vi "Folder fit WLC.vi"() -> ()   [LabVIEW 2014]
uses:
  SubVI/WLC-Fitting Cluster.ctl
  <vilib>/Utility/file.llb/Write To Spreadsheet File (DBL).vi
  <vilib>/Analysis/NI_AALBase.lvlib
panel:
  out "mean K":dbl format="%0.2f"
  out "Lp-Time":cluster{i32[], "best fit parameters":dbl[]}(graph)
  out "Lc-Time":cluster{i32[], "best fit parameters":dbl[]}(graph)
  out "median Lc":dbl format="%0.2f"
  out "median Lp":dbl format="%0.2f"
  in  "Save?":bool
  in  "Enum":T1(ring)
  out "STD Lc":dbl format="%0.2f"
  out "STD Lp":dbl format="%0.2f"
  in  "DataRecord type":enum32{"OneDirectionOnly?", "TwoSide Data"}(tab)=enum."TwoSide Data"
  out "OneDirectionOnly?":bool=TRUE
  in  "Fit \"+\"(RHS) ?":bool=TRUE
  in  "Fit One Side?":bool
  out "r^2 Array":dbl[](array[numeric])
  out "mean Lc":dbl format="%0.2f"
  out "mean Lp":dbl format="%0.2f"
  out "Lc array":dbl[](array[numeric])
  out "Lp array":dbl[](array[numeric])
  out "best fit parameters":dbl[][](array[numeric])
  in  "Fitting Cluster":T2={"cr (um)"=0.0, "yr (V)"=0.0, "trap height(nm)"=300.0, "bead radius(nm)"=515.0, "Length offset"=550.0, "Upper Force(pN)"=500.0, "cr shift (nm)"=0.0, "yr shift (mV)"=0.0, "LaserPower (mW)"=1000.0, "conversion factor (V/um)"=0.0, "Stiffness (pN/nm)"=0.0, "xDNA cut outside"=3000.0, "Lower Force(pN)"=5.0, "c for zbd"=0.002}
  in  "initial parameters (Lp,Lc) or (Lc,K)":dbl[](array[numeric])=[40.0, 1150.0]
  in  "Folder Path":path
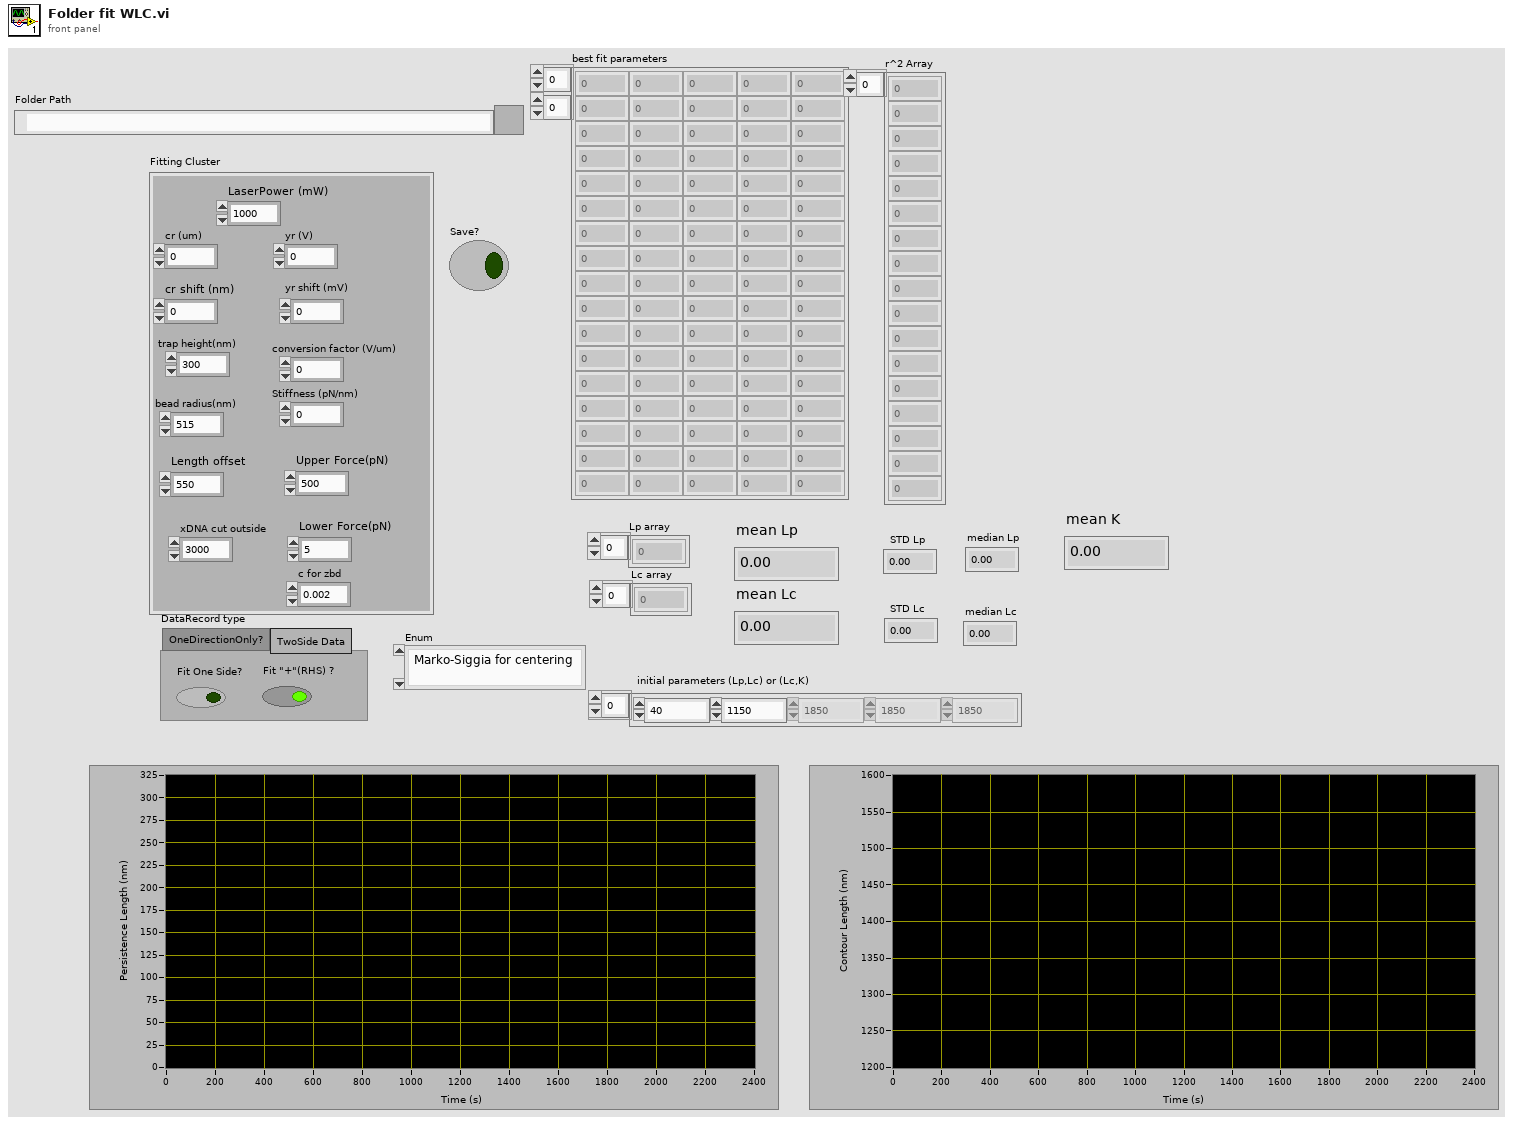
[diagram p1: front panel]
types:
  T1 = enum16{" Marko-Siggia for centering", "Marko-Siggia", "direct fit (Lp,Lc,K)", "fit K (Lp,Lc,K)", "eWLC (Lp=45,Lc,K)"}
  T2 = typedef "WLC-Fitting Cluster.ctl" = cluster{"cr (um)":dbl, "yr (V)":dbl, "trap height(nm)":dbl, "bead radius(nm)":dbl, "Length offset":dbl, "Upper Force(pN)":dbl, "cr shift (nm)":dbl, "yr shift (mV)":dbl, "LaserPower (mW)":dbl, "conversion factor (V/um)":dbl, "Stiffness (pN/nm)":dbl, "xDNA cut outside":dbl, "Lower Force(pN)":dbl, "c for zbd":dbl}
  T3 = cluster{"Time past (s)":i32[], "best fit parameters":dbl[]}
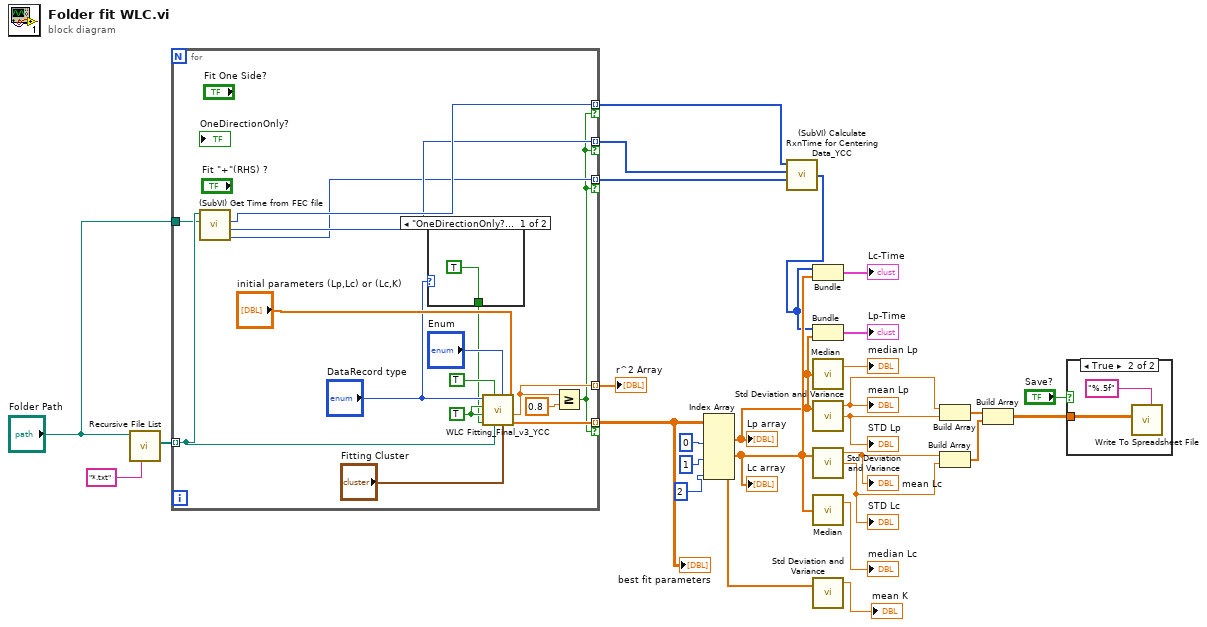
[diagram p0: block diagram]
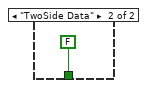
[diagram p3: hidden frame]
diagram:
  n1 = call <vilib>:"Recursive File List.vi"("pattern"="*.txt", "Folder Path"="Folder Path") -> ("All Files in Dir"=w27:path[])  [unwired: 5 in, 4 out]
  n2 = for {
    tunnel: w27 -> [w35] mode=indexing
    tunnel: [w41] -> w4 mode=indexing if=w30
    tunnel: [w39] -> w24 mode=indexing
    tunnel: "Folder Path" -> [w34]
    tunnel: [w33] -> w8 mode=indexing if=w30
    tunnel: [w32] -> w7 mode=indexing if=w30
    tunnel: [w31] -> w6 mode=indexing if=w30
    w44 = TRUE ("Ready to Fit")
    n3 = call "(SubVI) Get Time from FEC file.vi"("Folder path"=w34, "path"=w35) -> ("sec"=w31:i32, "min"=w32:i32, "hr"=w33:i32)  [unwired: 2 in, 1 out]
    n4 = case shown="\"OneDirectionOnly?\", Default" "DataRecord type" {
      tunnel: [TRUE ("T=Fit U or twoside\nF=Fit F") FALSE ("Save Calibrated Data?")] -> w29
      frame "OneDirectionOnly?", Default {
      }
      frame "TwoSide Data" {
      }
    }
    n5 = call "WLC Fitting_Final_v3_YCC.vi"("initial parameters (Lp,Lc) or (Lc,K)"="initial parameters (Lp,Lc) or (Lc,K)", "Fitting Cluster"="Fitting Cluster", "Enum"="Enum", "Load Stage-QPD data"=w35, "T=Fit U or twoside\nF=Fit F"=TRUE ("T=Fit U or twoside\nF=Fit F"), "F+U data?"=w29, "Finish Fitting"=w44, "Ready to Fit"=w44, "DataRecord type"="DataRecord type") -> ("best fit parameters"=w41:dbl[], "r^2"=w39:dbl)  [unwired: 1 in]
    n6 = Greater Or Equal?(x=w39, y=0.8) -> (x >= y?=w30:bool)
  }
  "best fit parameters" <- w4
  "r^2 Array" <- w24
  n7 = Index Array(array=w4, index (col) #1=0 ("disabled index (col)"), index (col) #2=1 ("disabled index (col)"), index (col) #3=2 ("disabled index (col)")) -> (element #1=w10:dbl[], element #2=w13:dbl[], element #3=w2:dbl[])  [unwired: 3 in]
  "Lp array" <- w10
  "Lc array" <- w13
  n8 = call "(SubVI) Calculate RxnTime for Centering Data_YCC.vi"("sec array"=w6, "min array"=w7, "hr array"=w8) -> ("Time past (s)"=w5:i32[])  [unwired: 3 in]
  n9 = Bundle("Time past (s)"=w5, "best fit parameters"=w13) -> (→"Lc-Time":T3)  [unwired: 1 in]
  n10 = Bundle("Time past (s)"=w5, "best fit parameters"=w10) -> (→"Lp-Time":T3)  [unwired: 1 in]
  n11 = call <vilib>:"Median.vi"("X"=w10) -> ("median"=→"median Lp":dbl)  [unwired: 1 out]
  n12 = call <vilib>:"Std Deviation and Variance.vi"("X"=w10) -> ("mean"=w23:dbl, "standard deviation"=w22:dbl)  [unwired: 1 in, 1 out]
  "mean Lp" <- w23
  "STD Lp" <- w22
  n13 = call <vilib>:"Std Deviation and Variance.vi"("X"=w13) -> ("mean"=w21:dbl, "standard deviation"=w20:dbl)  [unwired: 1 in, 1 out]
  "mean Lc" <- w21
  "STD Lc" <- w20
  n14 = call <vilib>:"Median.vi"("X"=w13) -> ("median"=→"median Lc":dbl)  [unwired: 1 out]
  n15 = call <vilib>:"Std Deviation and Variance.vi"("X"=w2) -> ("mean"=→"mean K":dbl)  [unwired: 1 in, 2 out]
  n16 = Build Array(w23, w22) -> (w19:dbl[])
  n17 = Build Array(w21, w20) -> (w18:dbl[])
  n18 = Build Array(w19, w18) -> (w17:dbl[][])
  n19 = case shown="True" "Save?" {
    tunnel: w17 -> [_ w48]
    frame False {
    }
    frame True {
      n20 = call-poly <vilib>:"Write To Spreadsheet File.vi"("format (%.3f)"="%.5f", "2D data"=w48) -> ()  [unwired: 6 in, 1 out]
    }
  }
